vi "Generic 1 Axis DAQmx AO Stage Engine.vi"(0 "Unique Notifier Name":string="Not a Name", 11 "DIO Lines":string[](array[string])) -> ()   [LabVIEW 2020]
uses:
  Stages Controls/Stage Notifier Element.ctl
  Stages Controls/Stage Actions.ctl
  Stages Controls/Stage Status.ctl
  <vilib>/DAQmx/write.llb/DAQmx Write (Analog DBL 1Chan 1Samp).vi
  <vilib>/DAQmx/create/channels.llb/DAQmx Create Channel (AO-Voltage-Basic).vi
  <vilib>/DAQmx/miscellaneous.llb/DAQmx Fill In Error Info.vi
panel:
  in  "Quit":bool
  in  "Home":bool
  in  "Get Position":bool
  in  "Position (µm)":dbl format="%#_4g"
  in  "Step Size (µm)":dbl format="%#_4g"
  in  "Up":bool
  in  "Down":bool
  # "Array Elements must be:\n\n1) AO Channel (e.g. Dev1/ao0)\n2) Max voltage\n3) Min voltage\n4) Volts/µm"
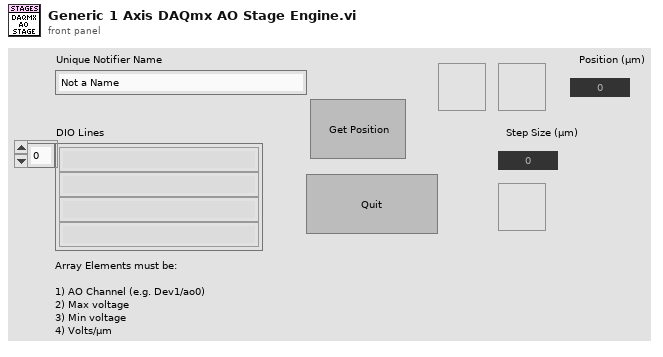
[diagram p1: front panel]
types:
  T1 = typedef "Stage Notifier Element.ctl" = cluster{"Action":T2, "Axis":bool[], "Setpoint":dbl[], "Velocity":dbl, "Cmd Recvd?":bool, "Position":dbl[], "Status":T3, "Misc":variant}
  T2 = typedef "Stage Actions.ctl" = enum16{"Get Position", "MVR", "MOVE", "HALT", "ONTARGET", "ERROR", "REFERENCE", "INIT", "VELOCITY", "STATUS", "EXIT", "HOME", "ZEROPOS", "NANOPOS", "ANALOG", "QUIT"}
  T3 = typedef "Stage Status.ctl" = enum16{"Error", "Abort", "Busy", "On Target"}
  T4 = enum32{"Invalid", "Standard", "Closed", "Hidden", "Minimized", "Maximized"}
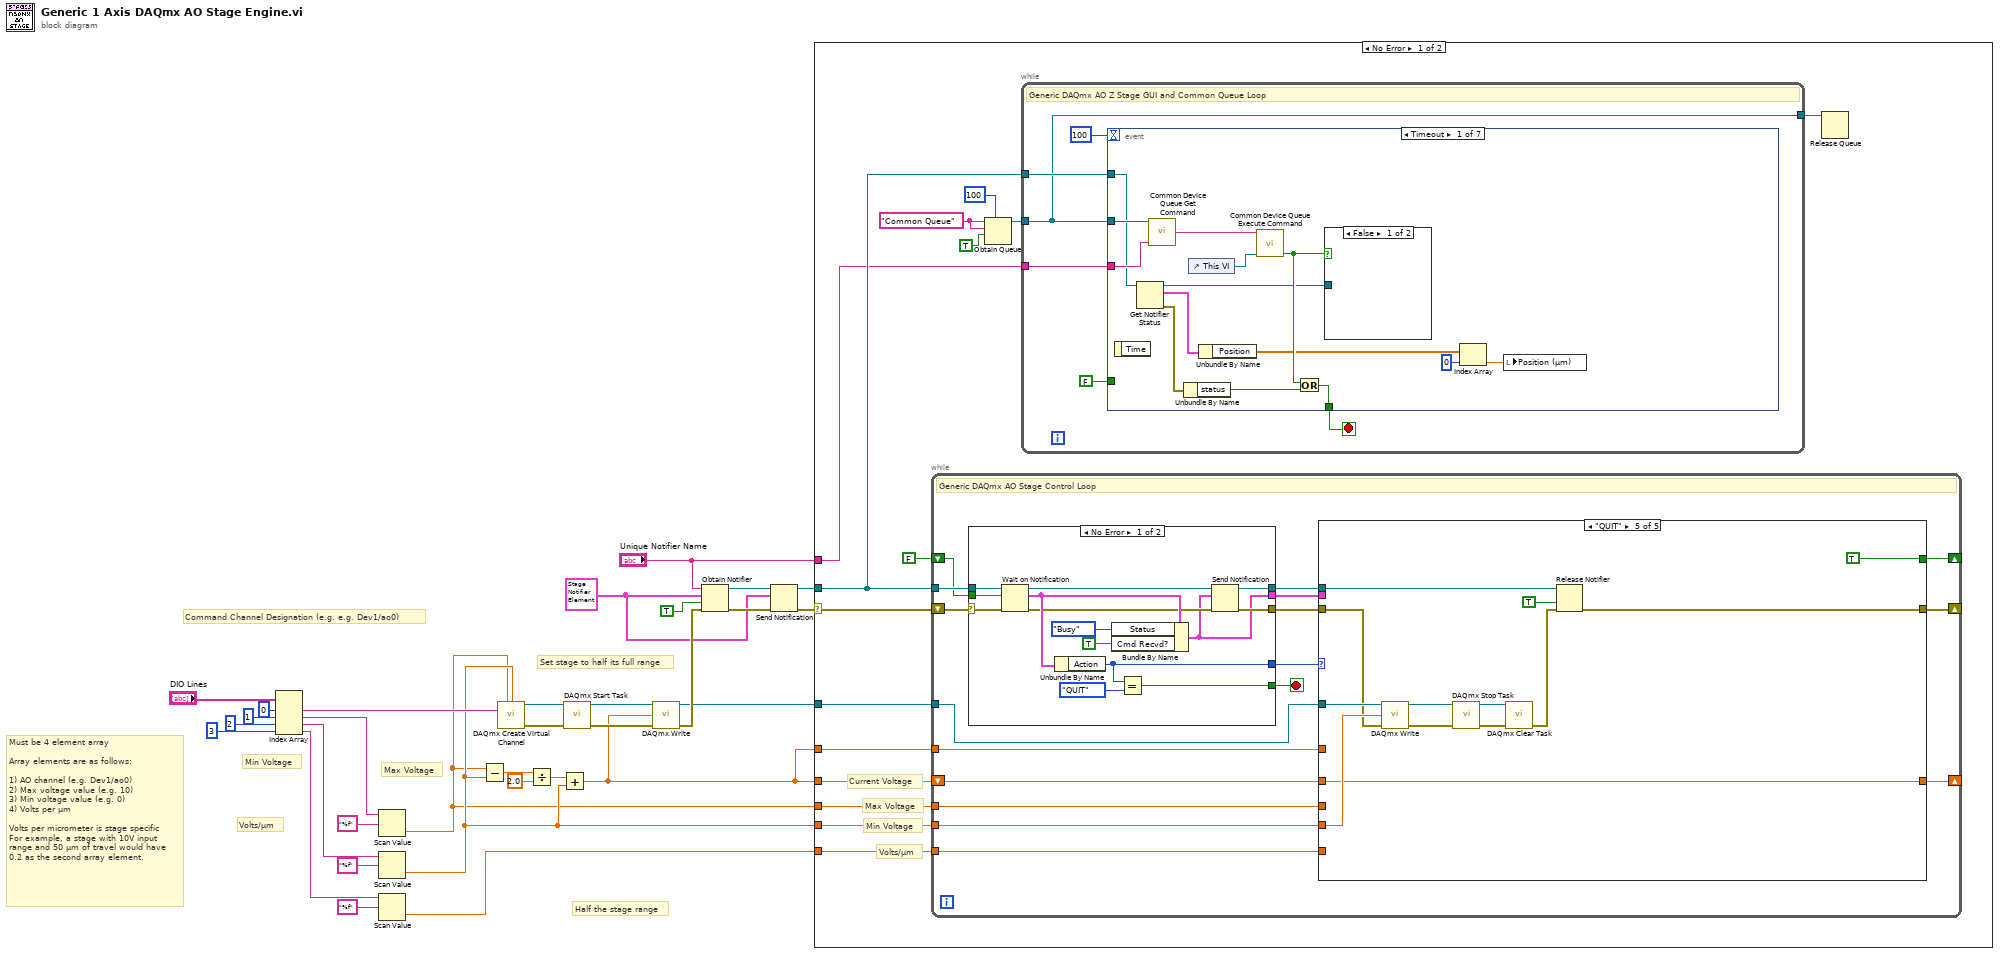
[diagram p0: block diagram]
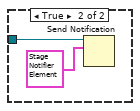
[diagram p2: hidden frame]
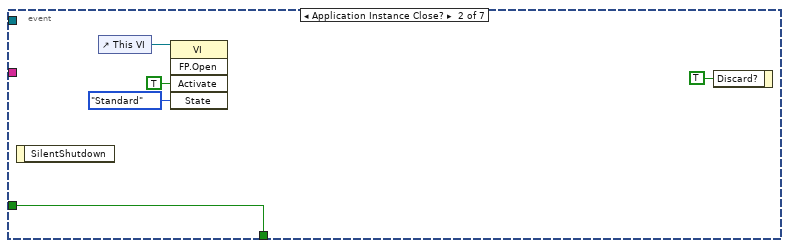
[diagram p3: hidden frame]
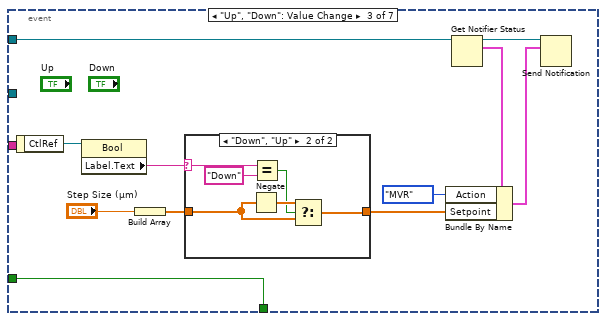
[diagram p4: hidden frame]
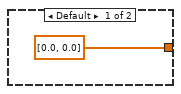
[diagram p5: hidden frame]
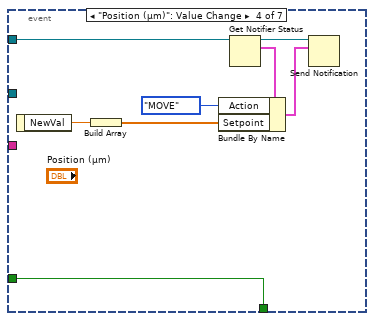
[diagram p6: hidden frame]
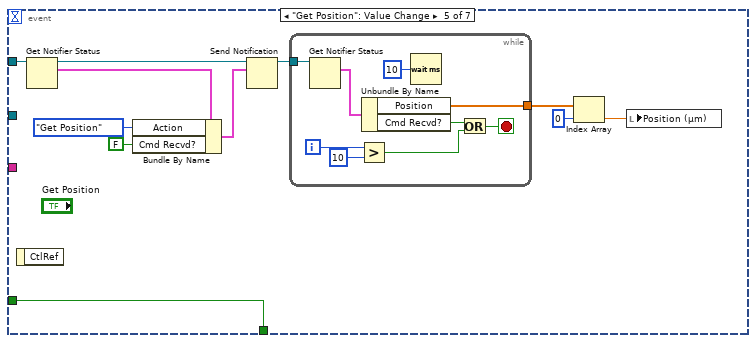
[diagram p7: hidden frame]
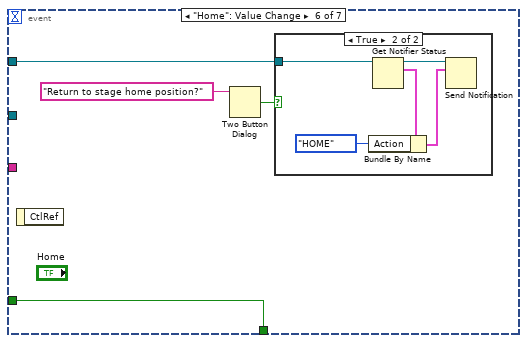
[diagram p8: hidden frame]
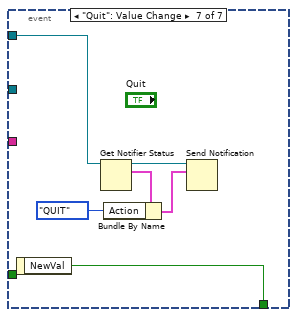
[diagram p10: hidden frame]
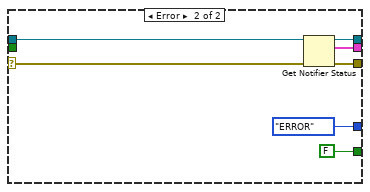
[diagram p11: hidden frame]
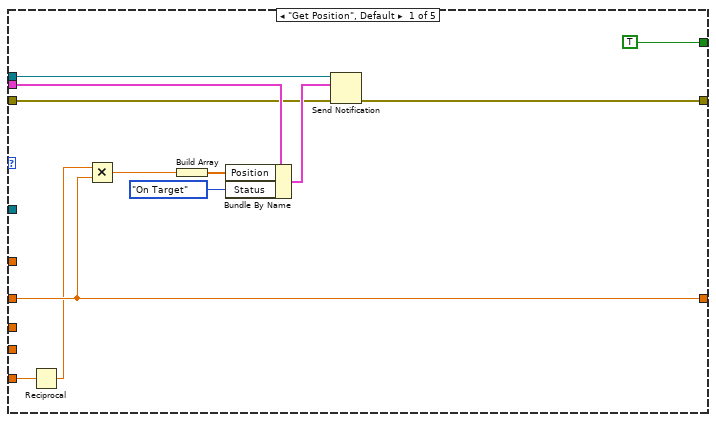
[diagram p12: hidden frame]
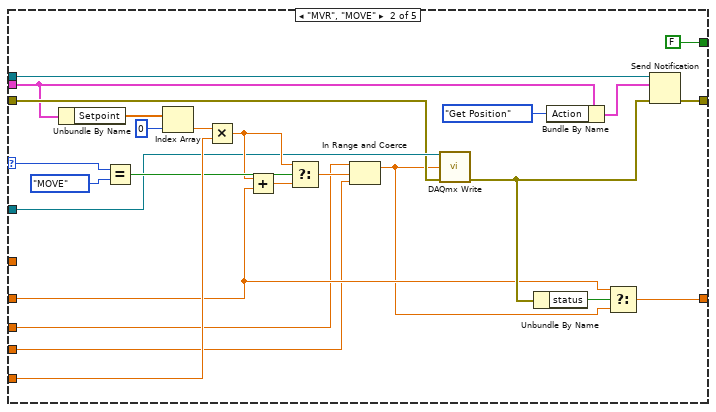
[diagram p13: hidden frame]
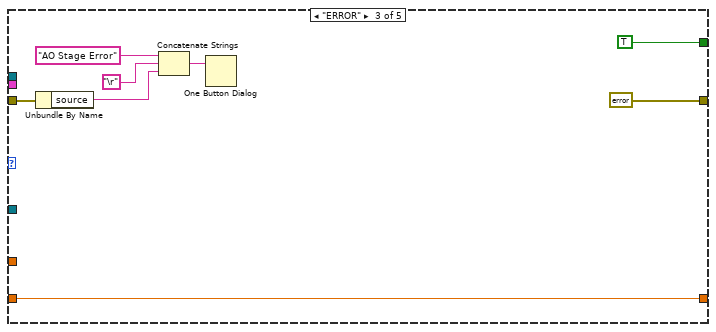
[diagram p14: hidden frame]
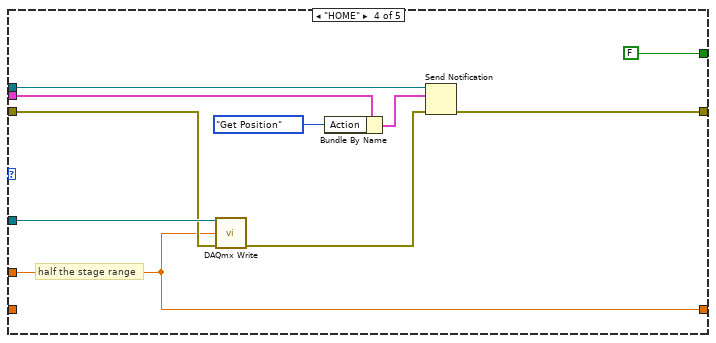
[diagram p15: hidden frame]
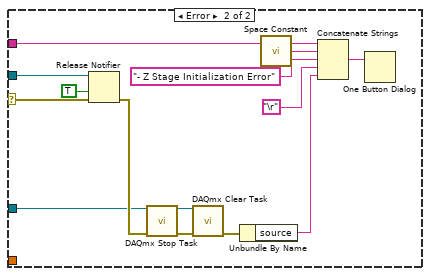
[diagram p16: hidden frame]
diagram:
  w2 = T1 {"Action"=enum."Get Position", "Axis"=[], "Setpoint"=[], "Velocity"=0.5, "Cmd Recvd?"=FALSE, "Position"=[], "Status"=enum."On Target", "Misc"=variant} ("Stage Status")
  # "Set stage to half its full range"
  # "Half the stage range"
  # "Volts/µm"
  # "Min Voltage"
  # "Max Voltage"
  # "Must be 4 element array\n\nArray elements are as follows:\n\n1) AO channel (e.g. Dev1/ao0)\n2) Max voltage value (e.g. 10)\n3) Min voltage value (e.g. 0)\n4) Volts per µm\n\nVolts per micrometer is stage specific\nFor example, a stage with 10V input\nrange and 50 µm of travel would have\n0.2 as the second array element."
  # "Command Channel Designation (e.g. e.g. Dev1/ao0)"
  n1 = Index Array(array="DIO Lines", index #1=0 ("index"), index #2=1 ("index"), index #3=2 ("index"), index #4=3 ("index")) -> (element #1=w25:string, element #2=w18:string, element #3=w17:string, element #4=w16:string)
  n2 = Scan Value(string=w18, format string="%f") -> (value=w1:dbl)  [unwired: 1 in, 1 out]
  n3 = Scan Value(string=w17, format string="%f") -> (value=w8:dbl)  [unwired: 1 in, 1 out]
  n4 = Scan Value(string=w16, format string="%f") -> (value=w9:dbl)  [unwired: 1 in, 1 out]
  n5 = Subtract(x=w1, y=w8) -> (x-y=w14:dbl)
  n6 = call-poly <vilib>:"DAQmx Create Virtual Channel.vi"("maximum value"=w1, "minimum value"=w8, "physical channels"=w25) -> ("task out"=w31:refnum<k21>, "error out"=w32:errorcluster)  [unwired: 6 in, 5 out]
  n7 = Divide(x=w14, y=2.0) -> (x/y=w12:dbl)
  n8 = Add(x=w12, y=w8) -> (x+y=w7:dbl)
  n9 = call <vilib>:"DAQmx Start Task.vi"("task/channels in"=w31, "error in"=w32) -> ("task out"=w28:refnum<k21>, "error out"=w29:errorcluster)  [unwired: 12 out]
  n10 = call-poly <vilib>:"DAQmx Write.vi"("task/channels in"=w28, "data"=w7, "error in"=w29) -> ("task out"=w10:refnum<k21>, "error out"=w15:errorcluster)  [unwired: 1 in, 10 out]
  n11 = Obtain Notifier(name (unnamed)="Unique Notifier Name", notification data type=w2, create if not found? (T)=TRUE, error in (no error)=w15) -> (notifier out=w6:refnum<notifier>, error out=w5:errorcluster)  [unwired: 1 out]
  n12 = Send Notification(notification=w2, notifier=w6, error in (no error)=w5) -> (notifier out=w3:refnum<notifier>, error out=w4:errorcluster)
  n13 = case shown="No Error" w4 {
    selector: w4 -> [w46 w243]
    tunnel: "Unique Notifier Name" -> [w35 w245]
    tunnel: w3 -> [w36 w244]
    tunnel: w10 -> [w47 w242]
    tunnel: w7 -> [w45 _]
    tunnel: w9 -> [w43 _]
    tunnel: w8 -> [w42 _]
    tunnel: w7 -> [w41 _]
    tunnel: w1 -> [w34 _]
    frame No Error {
      w39 = "Common Queue" ("Unique Notifier Name")
      # "Max Voltage"
      # "Current Voltage"
      # "Min Voltage"
      # "Volts/µm"
      n14 = while {
        tunnel: w36 -> [w152]
        tunnel: w47 -> [w138]
        shift-right: [w144] -> _
        shift-left: w45 -> [w145]
        shift-right: [w139] -> _
        shift-left: FALSE -> [w149]
        tunnel: w43 -> [w148]
        tunnel: w42 -> [w147]
        shift-right: [w146] -> _
        shift-left: w46 -> [w137]
        tunnel: w41 -> [w143]
        tunnel: w34 -> [w136]
        stop <- w151 stop-if-true
        # "Generic DAQmx AO Stage Control Loop"
        n15 = case shown="No Error" w137 {
          selector: w137 -> [w153 w171]
          tunnel: w152 -> [w166 w172]
          tunnel: [w164 FALSE] -> w151
          tunnel: [w163 Stage_Actions."ERROR" ("Action")] -> w150
          tunnel: w149 -> [w162 _]
          tunnel: [w158 w170] -> w142
          tunnel: [w157 w168] -> w141
          tunnel: [w155 w169] -> w140
          frame No Error {
            n16 = Wait on Notification(notifier=w166, ignore previous (F)=w162, error in (no error)=w153) -> (notifier out=w159:refnum<notifier>, notification=w161:T1, error out=w156:errorcluster)  [unwired: 1 in, 1 out]
            n17 = Unbundle By Name(w161) -> ("Action"=w163:T2)
            n18 = Bundle By Name(cluster=w161, "Status"=Stage_Status."Busy", "Cmd Recvd?"=TRUE) -> (w155:T1)
            n19 = Equal?(x=w163, y=Stage_Actions."QUIT") -> (x = y?=w164:bool)
            n20 = Send Notification(notification=w155, notifier=w159, error in (no error)=w156) -> (notifier out=w158:refnum<notifier>, error out=w157:errorcluster)
          }
          frame Error {
            n21 = Get Notifier Status(notifier=w172, error in (no error)=w171) -> (notifier out=w170:refnum<notifier>, current notification=w169:T1, error out=w168:errorcluster)  [unwired: 2 out]
          }
        }
        n22 = case shown="\"QUIT\"" w150 {
          selector: w150 -> [_ w210 _ _ _]
          tunnel: w148 -> [w178 w208 _ _ _]
          tunnel: w147 -> [_ w187 _ _ w240]
          tunnel: w142 -> [w185 w197 _ w223 w232]
          tunnel: w138 -> [_ w201 _ w228 w241]
          tunnel: w141 -> [w180 w200 w215 w227 w235]
          tunnel: [w179 w195 errorcluster {"status"=FALSE, "code"=0, "source"=""} ("Error") w220 w231] -> w146
          tunnel: w140 -> [w184 w199 _ w225 _]
          tunnel: w145 -> [w177 w191 w218 _ w230]
          tunnel: [w177 w190 w218 w226 w230] -> w144
          tunnel: w143 -> [_ _ _ w226 _]
          tunnel: [TRUE FALSE TRUE FALSE TRUE] -> w139
          tunnel: w136 -> [_ w186 _ _ _]
          frame "Get Position", Default {
            n23 = Reciprocal(x=w178) -> (1/x=w176:dbl)
            n24 = Multiply(x=w176, y=w177) -> (x*y=w175:dbl)
            n25 = Build Array(w175) -> (w182:dbl[])
            n26 = Bundle By Name(cluster=w184, "Position"=w182, "Status"=Stage_Status."On Target") -> (w183:T1)
            n27 = Send Notification(notification=w183, notifier=w185, error in (no error)=w180) -> (error out=w179:errorcluster)  [unwired: 1 out]
          }
          frame "MVR", "MOVE" {
            n28 = Unbundle By Name(w199) -> ("Setpoint"=w207:dbl[])
            n29 = Equal?(x=w210, y=Stage_Actions."MOVE") -> (x = y?=w204:bool)
            n30 = Index Array(array=w207, index=0) -> (element=w205:dbl)
            n31 = Multiply(x=w205, y=w208) -> (x*y=w202:dbl)
            n32 = Add(x=w202, y=w191) -> (x+y=w203:dbl)
            n33 = Select(t=w202, s=w204, f=w203) -> (s? t:f=w189:dbl)
            n34 = In Range and Coerce(upper limit=w186, x=w189, lower limit=w187) -> (coerced(x)=w188:dbl)  [unwired: 1 out]
            n35 = call-poly <vilib>:"DAQmx Write.vi"("task/channels in"=w201, "data"=w188, "error in"=w200) -> ("error out"=w193:errorcluster)  [unwired: 1 in, 11 out]
            n36 = Unbundle By Name(w193) -> ("status"=w192:bool)
            n37 = Bundle By Name(cluster=w199, "Action"=Stage_Actions."Get Position") -> (w196:T1)
            n38 = Select(t=w191, s=w192, f=w188) -> (s? t:f=w190:dbl)
            n39 = Send Notification(notification=w196, notifier=w197, error in (no error)=w193) -> (error out=w195:errorcluster)  [unwired: 1 out]
          }
          frame "ERROR" {
            n40 = Unbundle By Name(w215) -> ("source"=w212:string)
            n41 = Concatenate Strings("AO Stage Error" ("message"), "\r", w212) -> (w211:string)
            n42 = One Button Dialog(message=w211) -> ()  [unwired: 1 in, 1 out]
          }
          frame "HOME" {
            # "half the stage range"
            n43 = call-poly <vilib>:"DAQmx Write.vi"("task/channels in"=w228, "data"=w226, "error in"=w227) -> ("error out"=w222:errorcluster)  [unwired: 1 in, 11 out]
            n44 = Bundle By Name(cluster=w225, "Action"=Stage_Actions."Get Position") -> (w221:T1)
            n45 = Send Notification(notification=w221, notifier=w223, error in (no error)=w222) -> (error out=w220:errorcluster)  [unwired: 1 out]
          }
          frame "QUIT" {
            n46 = call-poly <vilib>:"DAQmx Write.vi"("task/channels in"=w241, "data"=w240, "error in"=w235) -> ("task out"=w239:refnum<k21>, "error out"=w237:errorcluster)  [unwired: 1 in, 10 out]
            n47 = call <vilib>:"DAQmx Stop Task.vi"("task/channels in"=w239, "error in"=w237) -> ("task out"=w238:refnum<k21>, "error out"=w236:errorcluster)  [unwired: 12 in]
            n48 = call <vilib>:"DAQmx Clear Task.vi"("task in"=w238, "error in"=w236) -> ("error out"=w233:errorcluster)  [unwired: 13 in]
            n49 = Release Notifier(notifier=w232, force destroy? (F)=TRUE, error in (no error)=w233) -> (error out=w231:errorcluster)  [unwired: 2 out]
          }
        }
      }
      n50 = Obtain Queue(max queue size (-1, unlimited)=100, name (unnamed)=w39, element data type=w39, create if not found? (T)=TRUE) -> (queue out=w40:refnum<queue>)  [unwired: 1 in, 2 out]
      n51 = while {
        tunnel: w40 -> [w48]
        tunnel: w35 -> [w51]
        tunnel: w36 -> [w52]
        tunnel: [w48] -> w33
        stop <- w50 stop-if-true
        # "Generic DAQmx AO Z Stage GUI and Common Queue Loop"
        n52 = event shown="[0] Timeout" {
          selector: _ -> [_ _ _ _ _ _ _]
          dyn-events: _ -> [_ _ _ _ _ _ _]
          timeout: 100 -> [_ _ _ _ _ _ _]
          tunnel: w48 -> [w61 _ _ _ _ _ _]
          tunnel: w52 -> [w58 _ w80 w98 w110 w121 w135]
          tunnel: w51 -> [w60 _ _ _ _ _ _]
          tunnel: [w59 w74 w83 w100 w111 w123 w131] -> w50
          tunnel: FALSE -> [_ w74 w83 w100 w111 w123 _]
          event Timeout {
            n53 = event-data() -> ()  [unwired: 1 in, 1 out]
            n54 = Get Notifier Status(notifier=w58) -> (notifier out=w62:refnum<notifier>, current notification=w57:T1, error out=w67:errorcluster)  [unwired: 1 in, 2 out]
            n55 = call "Common Device Queue Get Command.vi"("Common Queue"=w61, "Notifier Name"=w60) -> ("Command"=w66:string)  [unwired: 12 in, 1 out]
            n56 = Unbundle By Name(w67) -> ("status"=w64:bool)
            n57 = control-ref of="This VI"() -> (w65:refnum<vi>)
            n58 = Unbundle By Name(w57) -> ("Position"=w54:dbl[])
            n59 = call "Common Device Queue Execute Command.vi"("Common Command"=w66, "VI Refnum"=w65) -> ("Quit?"=w63:bool)  [unwired: 12 in, 1 out]
            n60 = Or(x=w63, y=w64) -> (x .or. y?=w59:bool)
            n61 = case shown="False" w63 {
              tunnel: w62 -> [_ w69]
              frame False {
              }
              frame True {
                n62 = Send Notification(notification=T1 {"Action"=enum."QUIT", "Axis"=[], "Setpoint"=[], "Velocity"=0.5, "Cmd Recvd?"=FALSE, "Position"=[], "Status"=enum."Error", "Misc"=variant} ("Stage Status"), notifier=w69) -> ()  [unwired: 1 in, 2 out]
              }
            }
            n63 = Index Array(array=w54, index=0) -> (element=w56:dbl)
            n64 = local write "Position (µm)"(w56) -> ()
          }
          event Application Instance Close? {
            n65 = event-data() -> ()  [unwired: 1 in, 1 out]
            n66 = control-ref of="This VI"() -> (w71:refnum<vi>)
            n67 = invoke class="VI" method="FP.Open"(reference=w71, "Activate"=TRUE ("Activate?"), "State"=T4."Standard") -> ()  [unwired: 2 in, 5 out]
            n68 = event-data("Discard?"=TRUE) -> ()  [unwired: 1 in, 1 out]
          }
          event "Up", "Down": Value Change {
            n69 = event-data() -> ("CtlRef"=w82:refnum<vi>)  [unwired: 1 in]
            n70 = property class="Bool"(reference=w82) -> ("Label.Text"=w85:string)  [unwired: 1 in, 2 out]
            n71 = Build Array("Step Size (µm)") -> (w84:dbl[])
            n72 = case shown="\"Down\", \"Up\"" w85 {
              selector: w85 -> [_ w92]
              tunnel: w84 -> [_ w89]
              tunnel: [dbl[] [0.0, 0.0] w88] -> w78
              frame Default {
              }
              frame "Down", "Up" {
                n73 = Negate(x=w89) -> (-x=w90:dbl[])
                n74 = Equal?(x=w92, y="Down") -> (x = y?=w87:bool)
                n75 = Select(t=w90, s=w87, f=w89) -> (s? t:f=w88:dbl[])
              }
            }
            n76 = Get Notifier Status(notifier=w80) -> (notifier out=w76:refnum<notifier>, current notification=w79:T1)  [unwired: 1 in, 3 out]
            n77 = Bundle By Name(cluster=w79, "Action"=Stage_Actions."MVR", "Setpoint"=w78) -> (w75:T1)
            n78 = Send Notification(notification=w75, notifier=w76) -> ()  [unwired: 1 in, 2 out]
          }
          event "Position (µm)": Value Change {
            n79 = event-data() -> ("NewVal"=w99:dbl)  [unwired: 1 in]
            n80 = Build Array(w99) -> (w95:dbl[])
            n81 = Get Notifier Status(notifier=w98) -> (notifier out=w97:refnum<notifier>, current notification=w96:T1)  [unwired: 1 in, 3 out]
            n82 = Bundle By Name(cluster=w96, "Action"=Stage_Actions."MOVE", "Setpoint"=w95) -> (w93:T1)
            n83 = Send Notification(notification=w93, notifier=w97) -> ()  [unwired: 1 in, 2 out]
          }
          event "Get Position": Value Change {
            n84 = event-data() -> ()  [unwired: 1 in, 1 out]
            n85 = Get Notifier Status(notifier=w110) -> (notifier out=w109:refnum<notifier>, current notification=w108:T1)  [unwired: 1 in, 3 out]
            n86 = Bundle By Name(cluster=w108, "Action"=Stage_Actions."Get Position", "Cmd Recvd?"=FALSE) -> (w105:T1)
            n87 = Send Notification(notification=w105, notifier=w109) -> (notifier out=w104:refnum<notifier>)  [unwired: 1 in, 1 out]
            n88 = while {
              tunnel: w104 -> [w120]
              tunnel: [w112] -> w103
              i -> [w116]
              stop <- w113 stop-if-true
              n89 = Get Notifier Status(notifier=w120) -> (current notification=w119:T1)  [unwired: 1 in, 4 out]
              n90 = Greater?(x=w116, y=10) -> (0:w114:bool)
              n91 = Unbundle By Name(w119) -> ("Position"=w112:dbl[], "Cmd Recvd?"=w115:bool)
              n92 = Wait (ms)(milliseconds to wait=u32 10) -> ()  [unwired: 1 out]
              n93 = Or(x=w115, y=w114) -> (x .or. y?=w113:bool)
            }
            n94 = Index Array(array=w103, index=0) -> (element=w101:dbl)
            n95 = local write "Position (µm)"(w101) -> ()
          }
          event "Home": Value Change {
            n96 = event-data() -> ()  [unwired: 1 in, 1 out]
            n97 = Two Button Dialog(message="Return to stage home position?") -> (T button?=w122:bool)  [unwired: 2 in]
            n98 = case shown="True" w122 {
              tunnel: w121 -> [_ w129]
              frame False {
              }
              frame True {
                n99 = Get Notifier Status(notifier=w129) -> (notifier out=w128:refnum<notifier>, current notification=w127:T1)  [unwired: 1 in, 3 out]
                n100 = Bundle By Name(cluster=w127, "Action"=Stage_Actions."HOME") -> (w126:T1)
                n101 = Send Notification(notification=w126, notifier=w128) -> ()  [unwired: 1 in, 2 out]
              }
            }
          }
          event "Quit": Value Change {
            n102 = event-data() -> ("NewVal"=w131:bool)  [unwired: 1 in]
            n103 = Get Notifier Status(notifier=w135) -> (notifier out=w134:refnum<notifier>, current notification=w133:T1)  [unwired: 1 in, 3 out]
            n104 = Bundle By Name(cluster=w133, "Action"=Stage_Actions."QUIT") -> (w132:T1)
            n105 = Send Notification(notification=w132, notifier=w134) -> ()  [unwired: 1 in, 2 out]
          }
        }
      }
      n106 = Release Queue(queue=w33) -> ()  [unwired: 2 in, 3 out]
    }
    frame Error {
      n107 = Release Notifier(notifier=w244, force destroy? (F)=TRUE, error in (no error)=w243) -> (error out=w252:errorcluster)  [unwired: 2 out]
      n108 = call <vilib>:"DAQmx Stop Task.vi"("task/channels in"=w242, "error in"=w252) -> ("task out"=w254:refnum<k21>, "error out"=w253:errorcluster)  [unwired: 12 in]
      n109 = call <vilib>:"DAQmx Clear Task.vi"("task in"=w254, "error in"=w253) -> ("error out"=w251:errorcluster)  [unwired: 13 out]
      n110 = Unbundle By Name(w251) -> ("source"=w246:string)
      n111 = call <vilib>:"Space Constant.vi"() -> ("String"=w249:string)
      n112 = Concatenate Strings(w245, w249, "- Z Stage Initialization Error" ("string"), "\r", w246) -> (w250:string)
      n113 = One Button Dialog(message=w250) -> ()  [unwired: 1 in, 1 out]
    }
  }
